vi "ep_Convert To U16 Waveforms Using RT Time.vi"(0 "DI data":u16[][](array[numeric]), 5 "sampling rate (Hz)":sgl=9600.0 format="%#.6g", 7 "RT controller time":timestamp, 9 "system info in":refnum<class "EP System Info.lvclass">, 11 "error in (no error)":errorcluster) -> (4 "digital data":waveform(u16)[](array[waveform]), 8 "interval time stamp":timestamp, 10 "system info out":refnum<class "EP System Info.lvclass">, 14 "interval length (s)":dbl, 15 "error out":errorcluster)   [LabVIEW 2013]
doc: "This VI builds voltage and current waveforms from input data, their sampling rate and RT controller time. Output waveforms contain basic measurement time interval of signal samples per channel, which represents 10-cycle time interval for a 50 Hz power system or 12-cycle time interval for a 60 Hz power system."
uses:
  <vilib>/addons/Electrical Power/PQ/Common/Classes/System Info/EP System Info.lvclass
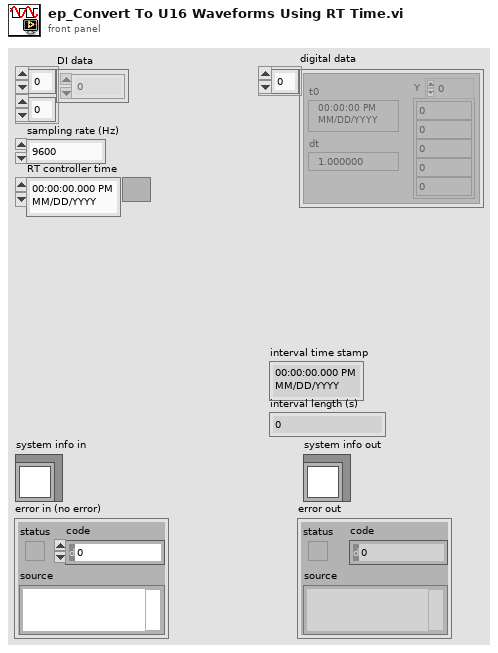
[diagram p1: front panel]
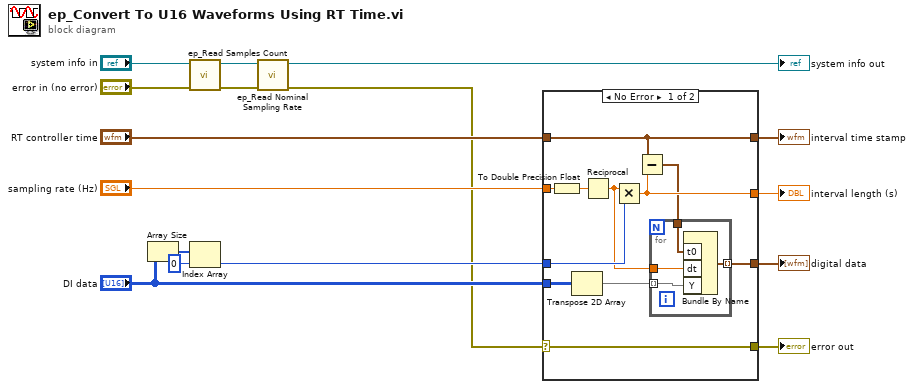
[diagram p0: block diagram]
diagram:
  n1 = Array Size(array="DI data") -> (size(s)=w11:i32[])
  n2 = call <vilib>:"ep_Read Samples Count.vi"("error in (no error)"="error in (no error)", "system info in"="system info in") -> ("error out"=w7:errorcluster, "system info out"=w6:refnum<class "EP System Info.lvclass">)  [unwired: 5 in, 3 out]
  n3 = Index Array(array=w11, index=0) -> (element=w5:i32)
  n4 = call <vilib>:"ep_Read Nominal Sampling Rate.vi"("error in (no error)"=w7, "system info in"=w6) -> ("error out"=w1:errorcluster, "system info out"=→"system info out":refnum<class "EP System Info.lvclass">)  [unwired: 7 in, 1 out]
  n5 = case shown="No Error" w1 {
    selector: w1 -> [w21 w32]
    tunnel: [w21 w32] -> w3
    tunnel: "sampling rate (Hz)" -> [w26 _]
    tunnel: "DI data" -> [w22 _]
    tunnel: "RT controller time" -> [w25 _]
    tunnel: [w23 _] -> w14
    tunnel: [w17 _] -> w13
    tunnel: [w25 _] -> w12
    tunnel: w5 -> [w24 _]
    frame No Error {
      n6 = To Double Precision Float(number=w26) -> (double precision float=w27:dbl)
      n7 = Transpose 2D Array(2D array=w22) -> (transposed array=w20:u16[][])
      n8 = Reciprocal(x=w27) -> (1/x=w18:dbl)
      n9 = Multiply(x=w18, y=w24) -> (x*y=w23:dbl)
      n10 = Subtract(x=w25, y=w23) -> (x-y=w19:timestamp)
      n11 = for {
        tunnel: w20 -> [w31] mode=indexing
        tunnel: w19 -> [w30]
        tunnel: w18 -> [w29]
        tunnel: [w28] -> w17 mode=indexing
        n12 = Bundle By Name("t0"=w30, "dt"=w29, "Y"=w31) -> (w28:waveform(u16))  [unwired: 1 in]
      }
    }
    frame Error {
    }
  }
  "digital data" <- w13
  "error out" <- w3
  "interval time stamp" <- w12
  "interval length (s)" <- w14
